vi "vms_putSample_CameraRotator.vi"(8 "error in (no error)":errorcluster, 11 "CameraRotator_Ctl":T1) -> (0 "error out":errorcluster, 2 "function return":i32, 3 "CameraRotator_Ctl out":T1)   [LabVIEW 2016, in "SALLV_vms.lvlib"]
doc: "int vms_shm_putSample_CameraRotatorLV(vms_CameraRotatorLV *CameraRotator_Ctl );"
uses:
  SALLV_vms.lvlib
  DataTypes/CameraRotator.ctl
  SALLV_vms.so
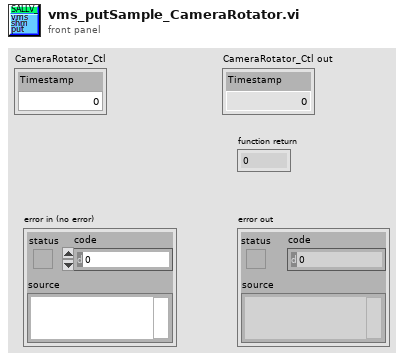
[diagram p1: front panel]
types:
  T1 = typedef "SALLV_vms.lvlib/CameraRotator.ctl" = cluster{"Timestamp":dbl}
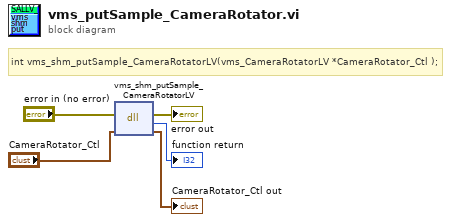
[diagram p0: block diagram]
diagram:
  # "int vms_shm_putSample_CameraRotatorLV(vms_CameraRotatorLV *CameraRotator_Ctl );"
  n1 = dll-call lib="opt/CODE/SALLV_vms/SALLV_vms.*" fn="vms_shm_putSample_CameraRotatorLV"(error in="error in (no error)", "CameraRotator_Ctl"="CameraRotator_Ctl") -> (error out=→"error out":errorcluster, →"function return":i32, "CameraRotator_Ctl"=→"CameraRotator_Ctl out":T1)  [unwired: 2 in, 1 out]
